vi "PID xcorrector.vi"(11 "Image width":dbl) -> (0 "Motor out":dbl, 3 "Good Enough?":bool)   [LabVIEW 2015]
uses:
  cogs.vi
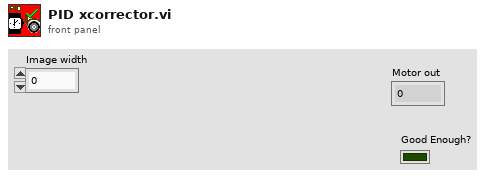
[diagram p1: front panel]
types:
  T1 = cluster{"Global Rectangle":cluster{"x1Left":i32, "y1Top":i32, "x2Right":i32, "y2Bottom":i32}, "Centroid":cluster{"x":sgl, "y":sgl}, "Object Size":u32, "Score":dbl}
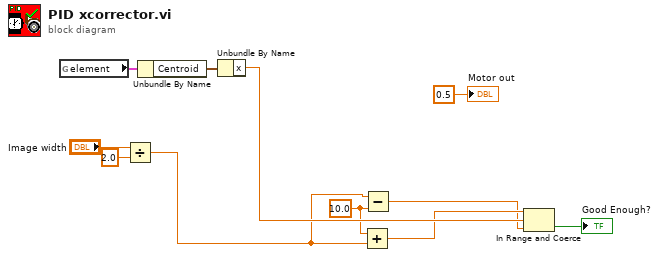
[diagram p0: block diagram]
diagram:
  w4 = sgl 10.0 ("x")
  n1 = global read "cogs.vi" "element"() -> (w11:T1)
  n2 = Divide(x="Image width", y=2.0) -> (x/y=w3:dbl)
  n3 = Unbundle By Name(w11) -> ("Centroid"=w10:cluster{"x":sgl, "y":sgl})
  n4 = Unbundle By Name(w10) -> ("x"=w5:sgl)
  n5 = Add(x=w4, y=w3) -> (x+y=w2:dbl)
  n6 = Subtract(x=w3, y=w4) -> (x-y=w1:dbl)
  n7 = In Range and Coerce(upper limit=w2, x=w5, lower limit=w1) -> (In Range?=→"Good Enough?":bool)  [unwired: 1 out]
  "Motor out" <- 0.5 ("Motor out")
